vi "End Group.vi"(8 "error in (no error)":errorcluster {"code" format="Error %.0f"}, 10 "Group":string, 11 "VIDoc Printer In":refnum<class "VIDoc Printer.lvclass">) -> (0 "error out":errorcluster {"code" format="Error %.0f"}, 3 "VIDoc Printer Out":refnum<class "VIDoc Printer.lvclass">)   [LabVIEW 2023, in "VIDoc Printer.lvlib" / "VIDoc Printer.lvclass"]
uses:
  VIDoc Printer.lvclass
  VIDoc Printer.lvclass/VIDoc Printer.ctl
  UI Interaction/Interface/UI Interaction.lvclass
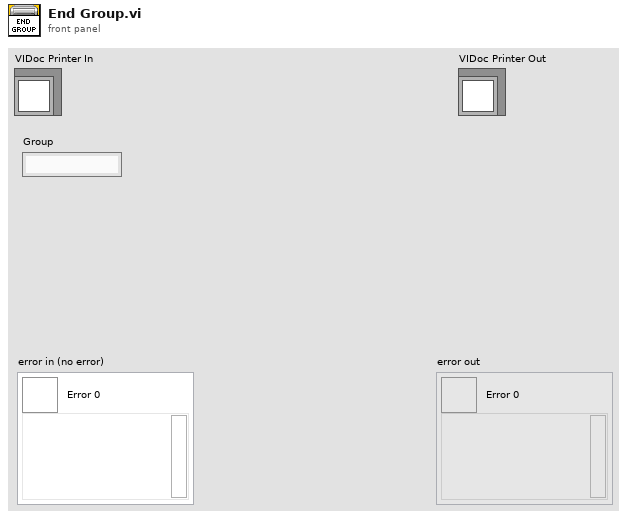
[diagram p1: front panel]
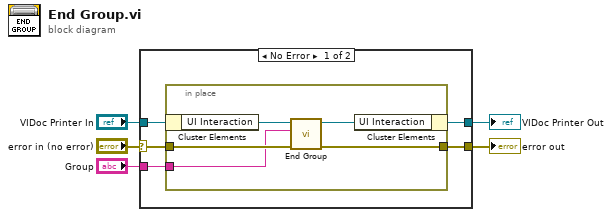
[diagram p0: block diagram]
diagram:
  n1 = case shown="No Error" "error in (no error)" {
    selector: "error in (no error)" -> [w8 w17]
    tunnel: [w7 w17] -> w4
    tunnel: [w10 w16] -> w2
    tunnel: "VIDoc Printer In" -> [w9 w16]
    tunnel: "Group" -> [w6 _]
    frame No Error {
      n2 = in-place {
        in-place-border: w8 -> [w13]
        in-place-border: [w11] -> w7
        in-place-border: w6 -> [w12]
        n3 = in-place-cluster #1(w9) -> ("UI Interaction"=w15:refnum<class "UI Interaction.lvclass">)
        n4 = call-dynamic "End Group.vi"("error in (no error)"=w13, "Group"=w12, "UI Interaction in"=w15) -> ("error out"=w11:errorcluster, "UI Interaction out"=w14:refnum<class "UI Interaction.lvclass">)  [unwired: 7 in]
        n5 = in-place-cluster #1("UI Interaction"=w14) -> (w10:refnum<class "VIDoc Printer.lvclass">)
      }
    }
    frame Error {
    }
  }
  "error out" <- w4
  "VIDoc Printer Out" <- w2
